vi "rus fit - write freqout file.vi"(4 "time points":dbl[](array[numeric]), 5 "Varshni win(relative)":dbl=1.2, 6 "to a file":string="2133_a", 7 "fit using":T1=enum."varshni", 8 "segments folder":path=path "C:/data/RUS/Experiment/ProbeTest/Probe8/SrKIr016/Sweep me baby 1/9w/2366_a.dat", 9 "freqout file":path=path "C:/data/RUS/Experiment/ProbeTest/Probe8/SrKIr016/Sweep me baby 1/9w/2366_a.dat", 10 "tfolder":T2={"tfolder path"=path "/snowfall/Users/arcadi/Desktop/Ultrasound/Experiment/YBCO_4/Round1/Sweep12/June_2011/062511/221.16400K_300_3100_001_062511.dat", "9folder path"=path "/snowfall/Users/arcadi/Desktop/Ultrasound/Experiment/YBCO_4/Round1/Sweep12/June_2011/062511/221.16400K_300_3100_001_062511.dat", "tfolder  -  file array"=[], "from index array"=[], "timestamp array"=[]}, 11 "lorentzian pts":T4[](array[typedef]) {"lorentzian"."z∞ (V)" format="%#_4p"; "lorentzian"."Q" format="%#_4p"; "lorentzian"."φ (rad)" format="%#_3p"; "lorentzian"."Γ (Hz)" format="%#_5p"; "lorentzian"."ω (Hz)" format="%#_9p"; "lorentzian"."A (VHz)" format="%#_3p"}) -> ()   [LabVIEW 2021]
uses:
  temperature sweep point.ctl
  lorentzian.ctl
  circle corners.ctl
  tfolder.ctl
  tfolder -- monotonic segment.ctl
  fit function selector control.ctl
  <vilib>/Utility/file.llb/Write To Spreadsheet File (string).vi
panel:
  in  "best fit parameters":dbl[](array[numeric])=[2165.147689441758, -122595126.26106773, 332463588576.80896]
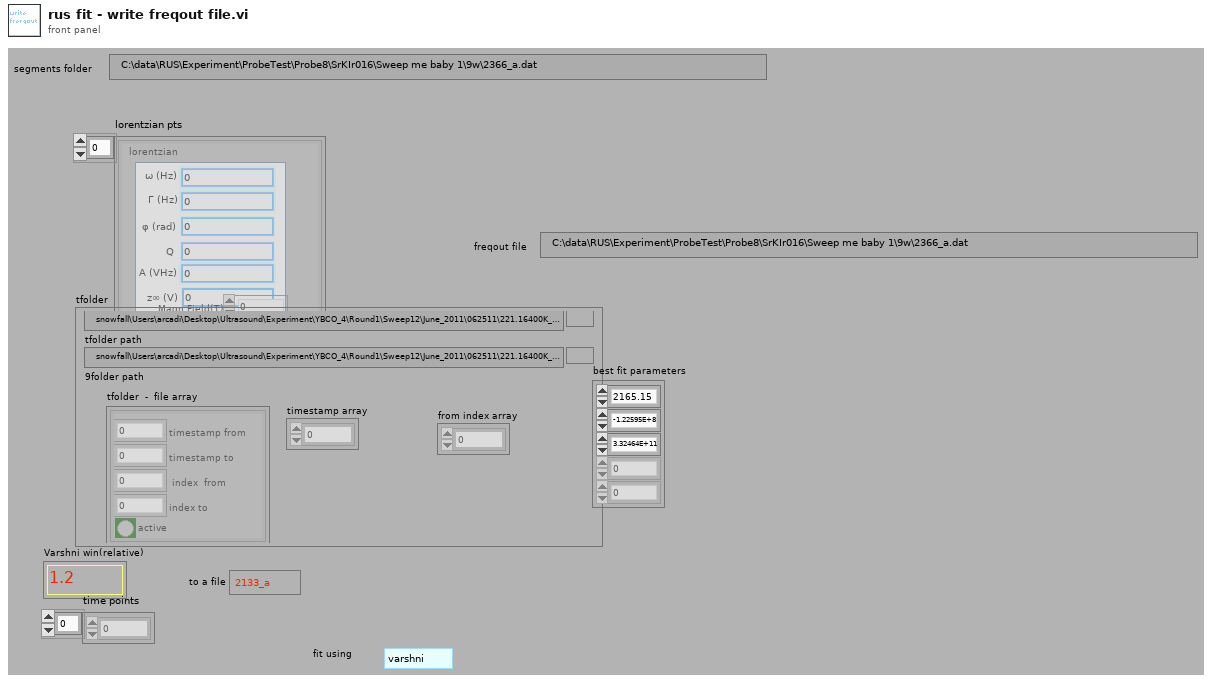
[diagram p1: front panel]
types:
  T1 = typedef "fit function selector control.ctl" = enum16{"linear", "varshni", "varshni5", "LogMinusT", "hyperbola", "einstein", "sine", "sine2theta", "cos2theta"}
  T2 = typedef "tfolder.ctl" = cluster{"tfolder path":path, "9folder path":path, "tfolder  -  file array":T3[], "from index array":i32[], "timestamp array":dbl[]}
  T3 = typedef "tfolder -- monotonic segment.ctl" = cluster{"timestamp from":dbl, "timestamp to":dbl, " index  from":i32, "index to":i32, "active":bool}
  T4 = typedef "temperature sweep point.ctl" = cluster{"temperature":dbl, "lorentzian":T5, "timestamp(min)":dbl, "timestamp":timestamp, "Magn Field(T)":dbl}
  T5 = typedef "lorentzian.ctl" = cluster{"A (VHz)":dbl, "ω (Hz)":dbl, "Γ (Hz)":dbl, "φ (rad)":dbl, "Q":dbl, "Norm  Ampl":dbl, "z∞ (V)":cdb, "4corners":T6}
  T6 = typedef "circle corners.ctl" = cluster{"z (-pi/2)":cdb, "z(inf)":cdb, "z (pi/2)":cdb, "z center":cdb, "z(0)":cdb, "radius":dbl}
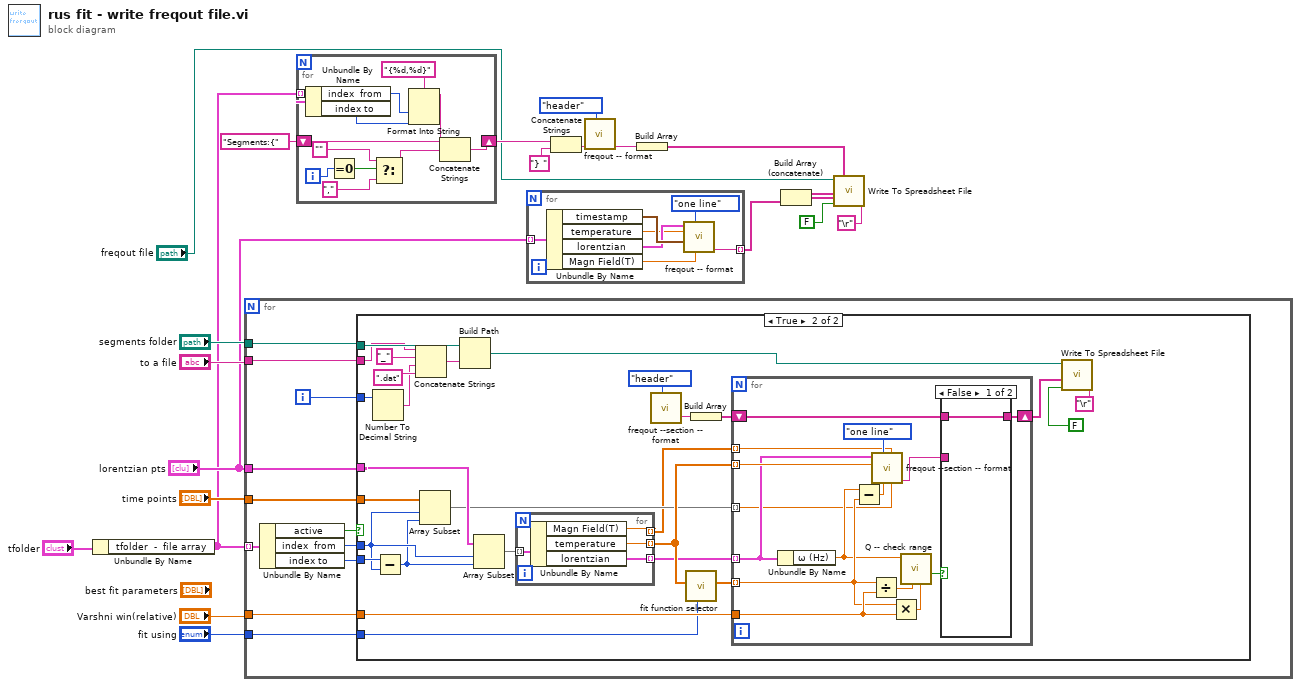
[diagram p0: block diagram]
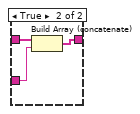
[diagram p3: hidden frame]
diagram:
  n1 = Unbundle By Name("tfolder") -> ("tfolder  -  file array"=w1:T3[])
  n2 = for {
    tunnel: w1 -> [w28] mode=indexing
    tunnel: "segments folder" -> [w31]
    tunnel: "to a file" -> [w30]
    tunnel: "lorentzian pts" -> [w26]
    tunnel: "Varshni win(relative)" -> [w24]
    tunnel: "time points" -> [w22]
    tunnel: "fit using" -> [w21]
    i -> [w29]
    n3 = Unbundle By Name(w28) -> ("active"=w23:bool, "index  from"=w25:i32, "index to"=w27:i32)
    n4 = case shown="True" w23 {
      tunnel: w31 -> [_ w56]
      tunnel: w30 -> [_ w55]
      tunnel: w29 -> [_ w54]
      tunnel: w27 -> [_ w51]
      tunnel: w26 -> [_ w50]
      tunnel: w25 -> [_ w39]
      tunnel: w24 -> [_ w45]
      tunnel: w22 -> [_ w40]
      tunnel: w21 -> [_ w36]
      frame False {
      }
      frame True {
        n5 = Number To Decimal String(number=w54) -> (decimal integer string=w52:string)  [unwired: 1 in]
        n6 = Subtract(x=w51, y=w39) -> (x-y=w38:i32)
        n7 = Concatenate Strings(w55, "_" ("name or relative path"), w52, ".dat" ("name or relative path")) -> (w57:string)
        n8 = Array Subset(array=w40, index=w39, length=w38) -> (w37:dbl[])
        n9 = Build Path(base path=w56, name or relative path=w57) -> (appended path=w47:path)
        n10 = Array Subset(array=w50, index=w39, length=w38) -> (w42:T4[])
        n11 = for {
          tunnel: w42 -> [w81] mode=indexing
          tunnel: [w80] -> w41 mode=indexing
          tunnel: [w79] -> w33 mode=indexing
          tunnel: [w78] -> w32 mode=indexing
          n12 = Unbundle By Name(w81) -> ("Magn Field(T)"=w78:dbl, "temperature"=w80:dbl, "lorentzian"=w79:T5)
        }
        n13 = call "freqout --section -- format.vi"("freqout action"=enum16{"header", "one line", "one"}."header") -> ("output string"=w35:string)  [unwired: 10 in]
        n14 = call "fit function selector.vi"("fit using"=w36, "temperature"=w41) -> ("freq out"=w46:dbl[])  [unwired: 7 in, 2 out]
        n15 = Build Array(w35) -> (w43:string[])
        n16 = for {
          tunnel: w46 -> [w67] mode=indexing
          shift-right: [w69] -> w44
          shift-left: w43 -> [w70]
          tunnel: w45 -> [w68]
          tunnel: w41 -> [w63] mode=indexing
          tunnel: w37 -> [w60] mode=indexing
          tunnel: w33 -> [w62] mode=indexing
          tunnel: w32 -> [w59] mode=indexing
          n17 = Unbundle By Name(w62) -> ("ω (Hz)"=w66:dbl)
          n18 = Subtract(x=w66, y=w67) -> (x-y=w61:dbl)
          n19 = Divide(x=w67, y=w68) -> (x/y=w72:dbl)
          n20 = call "freqout --section -- format.vi"("time (min)"=w60, "Magn Field (T)"=w59, "delta freq"=w61, "freqout action"=enum16{"header", "one line", "one"}."one line", "temperature"=w63, "lorentzian"=w62) -> ("output string"=w64:string)  [unwired: 5 in]
          n21 = Multiply(x=w67, y=w68) -> (x*y=w73:dbl)
          n22 = call "Q -- check range.vi"("upper"=w73, "lower"=w72, "number"=w66) -> ("in range?"=w71:bool)  [unwired: 4 in, 4 out]
          n23 = case shown="False" w71 {
            tunnel: w70 -> [w74 w77]
            tunnel: [w74 w76] -> w69
            tunnel: w64 -> [_ w75]
            frame False {
            }
            frame True {
              n24 = Build Array (concatenate)(w77, w75) -> (w76:string[])
            }
          }
        }
        n25 = call-poly <vilib>:"Write To Spreadsheet File.vi"("delimiter (\\t)"="\r", "append to file? (new file:F)"=FALSE, "1D data"=w44, "file path (dialog if empty)"=w47) -> ()  [unwired: 4 in, 1 out]
      }
    }
  }
  n26 = for {
    shift-right: [w91] -> w17
    shift-left: "Segments:{" -> [w92]
    tunnel: w1 -> [w93] mode=indexing
    i -> [w87]
    n27 = Unbundle By Name(w93) -> ("index  from"=w89:i32, "index to"=w88:i32)
    n28 = Equal To 0?(x=w87) -> (x = 0?=w86:bool)
    n29 = Select(t="", s=w86, f=",") -> (s? t:f=w82:string)
    n30 = Format Into String(format string="{%d,%d}", w89, w88) -> (resulting string=w83:string)  [unwired: 2 in, 1 out]
    n31 = Concatenate Strings(w92, w82, w83) -> (w91:string)
  }
  n32 = for {
    tunnel: "lorentzian pts" -> [w100] mode=indexing
    tunnel: [w95] -> w7 mode=indexing
    n33 = Unbundle By Name(w100) -> ("timestamp"=w98:timestamp, "temperature"=w96:dbl, "lorentzian"=w97:T5, "Magn Field(T)"=w94:dbl)
    n34 = call "freqout -- format.vi"("Magn Field (T)"=w94, "freqout action"=enum16{"header", "one line", "one"}."one line", "timestamp"=w98, "temperature"=w96, "lorentzian"=w97) -> ("output string"=w95:string)  [unwired: 6 in]
  }
  n35 = Concatenate Strings(w17, "} ") -> (w3:string)
  n36 = call "freqout -- format.vi"("freqout action"=enum16{"header", "one line", "one"}."header", "segments string"=w3) -> ("output string"=w2:string)  [unwired: 9 in]
  n37 = Build Array(w2) -> (w6:string[])
  n38 = Build Array (concatenate)(w6, w7) -> (w5:string[])
  n39 = call-poly <vilib>:"Write To Spreadsheet File.vi"("delimiter (\\t)"="\r", "append to file? (new file:F)"=FALSE, "1D data"=w5, "file path (dialog if empty)"="freqout file") -> ()  [unwired: 4 in, 1 out]
